vi "Set Config Value.vi"(8 "error in (no error)":errorcluster, 9 "Value":string, 10 "Config Key":string, 11 "Device in":refnum<class "Device.lvclass">) -> (0 "error out":errorcluster, 3 "Device out":refnum<class "Device.lvclass">)   [LabVIEW 2020, in "HAL.lvlib" / "Device.lvclass"]
uses:
  Device.lvclass
  Device.lvclass/Device.ctl
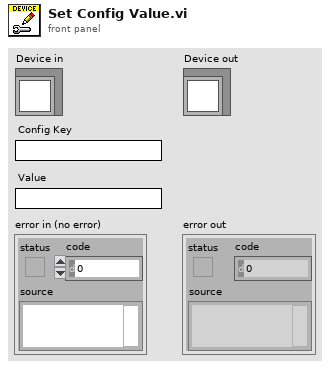
[diagram p1: front panel]
types:
  T1 = typedef "HAL.lvlib/Device.lvclass/Ref Data.ctl" = cluster{"Config Keys":string[], "Config Values":string[], "Cal Expires":timestamp, "Name":string, "Comment":string, "State":T2, "Error":errorcluster}
  T2 = typedef "HAL.lvlib/Device.lvclass/Device State.ctl" = enum16{"Uninitialized", "Initialized", "Configured", "Running", "Error"}
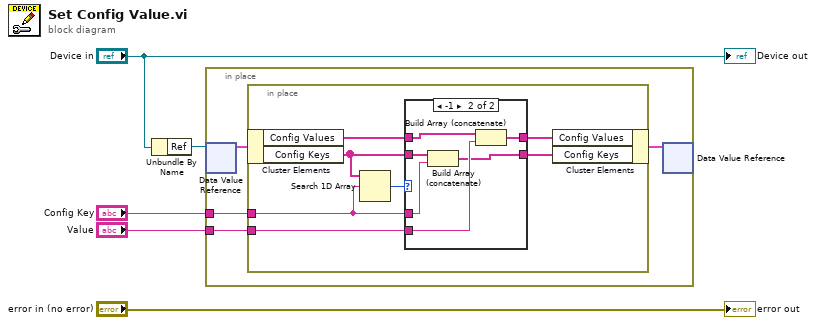
[diagram p0: block diagram]
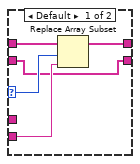
[diagram p2: hidden frame]
diagram:
  n1 = Unbundle By Name("Device in") -> ("Ref"=w4:refnum<data-value>)
  n2 = in-place {
    in-place-border: "Config Key" -> [w7]
    in-place-border: "Value" -> [w6]
    n3 = in-place-dvr #1(w4) -> (w9:T1)  [unwired: 1 out]
    n4 = in-place {
      in-place-border: w7 -> [w11]
      in-place-border: w6 -> [w12]
      n5 = in-place-cluster #2(w9) -> ("Config Values"=w14:string[], "Config Keys"=w16:string[])
      n6 = Search 1D Array(1D array=w16, element=w11) -> (index of element=w15:i32)  [unwired: 1 in]
      n7 = case shown="-1" w15 {
        selector: w15 -> [w20 _]
        tunnel: w16 -> [w17 w24]
        tunnel: w14 -> [w21 w27]
        tunnel: [w17 w22] -> w13
        tunnel: w12 -> [w19 w25]
        tunnel: w11 -> [_ w23]
        tunnel: [w18 w26] -> w10
        frame Default {
          n8 = Replace Array Subset(array=w21, new element=w19, index=w20) -> (w18:string[])
        }
        frame -1 {
          n9 = Build Array (concatenate)(w24, w23) -> (w22:string[])
          n10 = Build Array (concatenate)(w27, w25) -> (w26:string[])
        }
      }
      n11 = in-place-cluster #2("Config Values"=w10, "Config Keys"=w13) -> (w8:T1)
    }
    n12 = in-place-dvr #1(w8) -> ()  [unwired: 2 out]
  }
  "error out" <- "error in (no error)"
  "Device out" <- "Device in"
